vi "Save Image.vi"(8 "error in":errorcluster, 9 "Export Style":enum32{"Raw", "Graph", "Gray"}(radio), 10 "Export Name":string, 11 "Base Graph in":refnum<class "Base Graph.lvclass">) -> (0 "error out":errorcluster, 3 "Base Graph out":refnum<class "Base Graph.lvclass">)   [LabVIEW 2023, in "Base Graph.lvclass"]
uses:
  Base Graph.lvclass
  Base Graph.lvclass/Base Graph.ctl
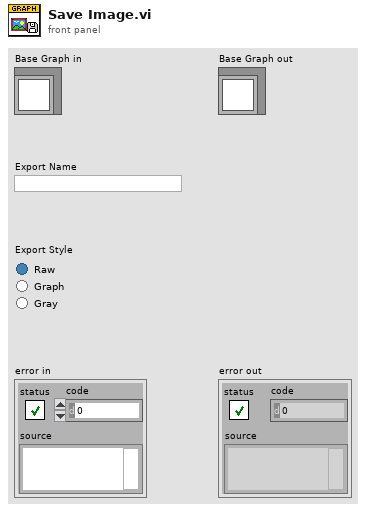
[diagram p1: front panel]
types:
  T1 = typedef "IMAQ Image.ctl" = refnum<image>
  T2 = typedef "imagedata.ctl" = cluster{"image type":i32, "image depth":i32, "image":u8[], "mask":u8[], "colors":u32[], "Rectangle":cluster{"left":i16, "top":i16, "right":i16, "bottom":i16}}
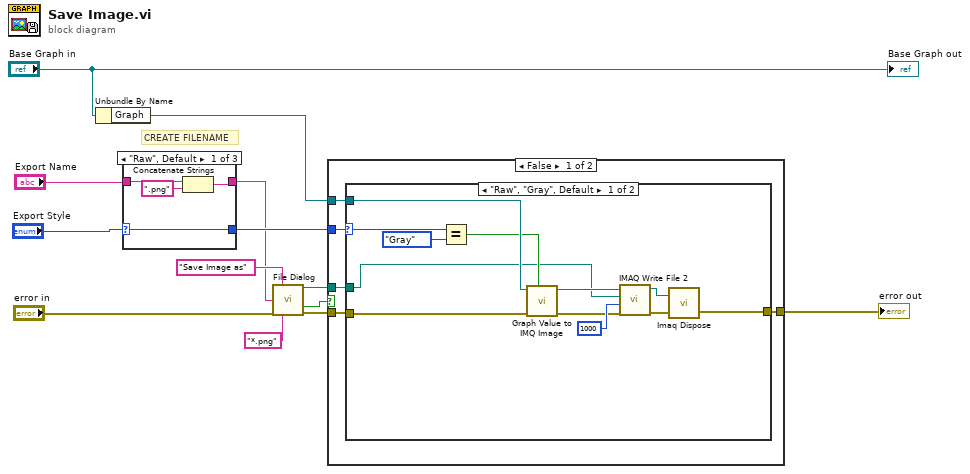
[diagram p0: block diagram]
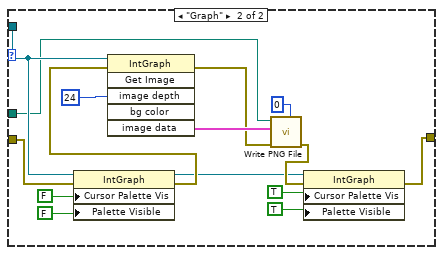
[diagram p2: hidden frame]
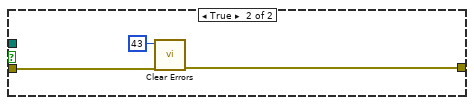
[diagram p3: hidden frame]
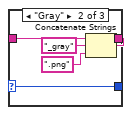
[diagram p4: hidden frame]
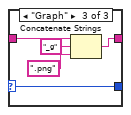
[diagram p5: hidden frame]
diagram:
  # "CREATE FILENAME"
  n1 = Unbundle By Name("Base Graph in") -> ("Graph"=w1:refnum<vi>)
  n2 = case shown="\"Raw\", Default" "Export Style" {
    selector: "Export Style" -> [w17 w20 w27]
    tunnel: [w17 w20 w27] -> w8
    tunnel: "Export Name" -> [w16 w22 w26]
    tunnel: [w14 w21 w23] -> w3
    frame "Raw", Default {
      n3 = Concatenate Strings(w16, ".png" ("string")) -> (w14:string)
    }
    frame "Gray" {
      n4 = Concatenate Strings(w22, "_gray" ("string"), ".png" ("string")) -> (w21:string)
    }
    frame "Graph" {
      n5 = Concatenate Strings(w26, "_g" ("string"), ".png" ("string")) -> (w23:string)
    }
  }
  n6 = call "File Dialog"("prompt"="Save Image as", "default name"=w3, "error in"="error in", "pattern (all files)"="*.png") -> ("selected path"=w2:path, "cancelled"=w4:bool, "error out"=w5:errorcluster)  [unwired: 8 in, 1 out]
  n7 = case shown="False" w4 {
    tunnel: [w32 w61] -> w12
    tunnel: w8 -> [w31 _]
    tunnel: w1 -> [w30 _]
    tunnel: w5 -> [w29 w62]
    tunnel: w2 -> [w28 _]
    frame False {
      n8 = case shown="\"Raw\", \"Gray\", Default" w31 {
        selector: w31 -> [w36 _]
        tunnel: w29 -> [w37 w49]
        tunnel: [w41 w46] -> w32
        tunnel: w30 -> [w38 w48]
        tunnel: w28 -> [w33 w47]
        frame "Raw", "Gray", Default {
          n9 = Equal?(x=w36, y=enum32{"Raw", "Graph", "Gray"}."Gray") -> (x = y?=w34:bool)
          n10 = call "Graph Value to IMQ Image.vi"("Gray?"=w34, "error in"=w37, "Intensity Graph Refnum"=w38) -> ("error out"=w39:errorcluster, "Image Out"=w44:T1)  [unwired: 7 in]
          n11 = call-poly "IMAQ Write File 2"("error in (no error)"=w39, "Image Quality"=u32 1000, "File Path"=w33, "Image"=w44) -> ("error out"=w42:errorcluster, "Image Out (duplicate)"=w43:T1)  [unwired: 6 in]
          n12 = call "Imaq Dispose"("Image"=w43, "error in (no error)"=w42) -> ("error out"=w41:errorcluster)  [unwired: 4 in]
        }
        frame "Graph" {
          n13 = property class="IntGraph"(reference=w48, error in=w49, "Cursor Palette Vis"=FALSE ("Cursor Legend Visible"), "Palette Visible"=FALSE ("Palette:Visible")) -> (reference out=w53:refnum<vi>, error out=w56:errorcluster)
          n14 = invoke class="IntGraph" method="Get Image"(reference=w48, error in=w56, "image depth"=24 ("Image Depth")) -> (error out=w57:errorcluster, "image data"=w58:T2)  [unwired: 3 in, 4 out]
          n15 = call <vilib>:"Write PNG File.vi"("compression (default)"=0, "error in (no error)"=w57, "image data"=w58, "path to PNG file"=w47) -> ("error out"=w54:errorcluster)  [unwired: 6 in, 1 out]
          n16 = property class="IntGraph"(reference=w53, error in=w54, "Cursor Palette Vis"=TRUE ("Cursor Legend Visible"), "Palette Visible"=TRUE ("Palette:Visible")) -> (error out=w46:errorcluster)  [unwired: 1 out]
        }
      }
    }
    frame True {
      n17 = call <vilib>:"Clear Errors.vi"("error in (no error)"=w62, "specific error code to clear (0: all)"=43) -> ("error out"=w61:errorcluster)  [unwired: 4 in, 1 out]
    }
  }
  "error out" <- w12
  "Base Graph out" <- "Base Graph in"
